vi "Is Error Vi.vi"(11 "Vi Name":string) -> (2 "Error Vi?":bool, 3 "Error Name":string)   [LabVIEW 2021, in "TAF Proj Document Type.lvlib" / "Project Parser.lvlib"]
uses:
  <vilib>/Wovalab/AntiDoc/Document Type/Add-ons/LabVIEW TAF Project/Project Parser/Project Parser.lvlib
  <vilib>/regexp/Match Regular Expression.xnode
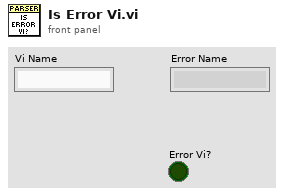
[diagram p1: front panel]
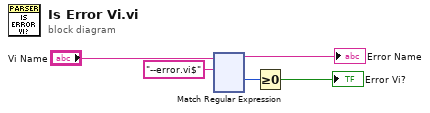
[diagram p0: block diagram]
diagram:
  n1 = xnode "Match Regular Expression"("input string"="Vi Name", "regular expression"="--error.vi$") -> ("before match"=→"Error Name":string, "offset past match"=w2:i32)  [unwired: 4 in, 3 out]
  n2 = Greater Or Equal To 0?(x=w2) -> (x >= 0?=→"Error Vi?":bool)
